vi "ADS1256 Init.vi"(9 "pConfig":T1, 10 "Channel":i8, 11 "DevIndex":i32) -> (3 "function return":i32)   [LabVIEW 2010, in "usb2ads1256.lvlib"]
doc: "int WINAPI ADS1256_Init(int DevIndex,char Channel,ADS1256_CONFIG *pConfig);"
uses:
  usb2ads1256.lvlib
  USB2XXX.dll
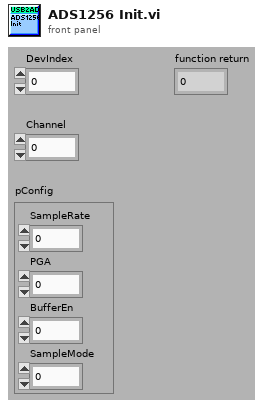
[diagram p1: front panel]
types:
  T1 = cluster{"SampleRate":u16, "PGA":u8, "BufferEn":u8, "SampleMode":u32}
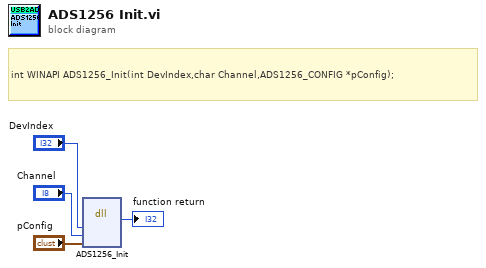
[diagram p0: block diagram]
diagram:
  # "int WINAPI ADS1256_Init(int DevIndex,char Channel,ADS1256_CONFIG *pConfig);"
  n1 = dll-call lib="F:/OtherWork/STM32/USB2XXX_Example/trunk/Labview/PublicFiles/usb2ads1256/USB2XXX.*" fn="ADS1256_Init"("DevIndex"="DevIndex", "Channel"="Channel", "pConfig"="pConfig") -> (→"function return":i32)  [unwired: 6 in, 2 out]
